vi "Initialize Root.vi"(6 "RootQueueName":string, 8 "error in (no error)":errorcluster caption="错误输入（无错误）", 9 "CurrentVi*":refnum<vi>, 10 "RootPanel*":refnum<vi>, 11 "PanelRootNode 输入":refnum<class "PanelRootNode.lvclass"> caption="DNL_LabVIEW Object in") -> (0 "error out":errorcluster caption="错误输出", 2 "SelfNode*":refnum<data-value>)   [LabVIEW 2013, in "PanelRootNode.lvclass"]
uses:
  PanelRootNode.lvclass
  PanelRootNode.lvclass/PanelRootNode.ctl
  PanelDataNode/PanelDataNode.lvclass/PanelDataNode.ctl
  PanelDataNode/PanelDataNode.lvclass
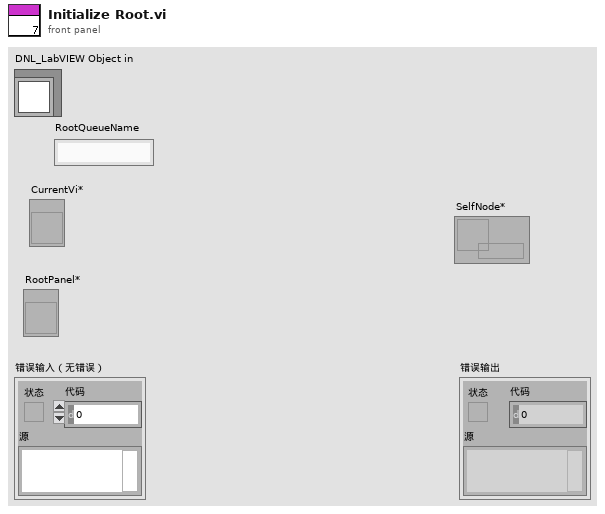
[diagram p1: front panel]
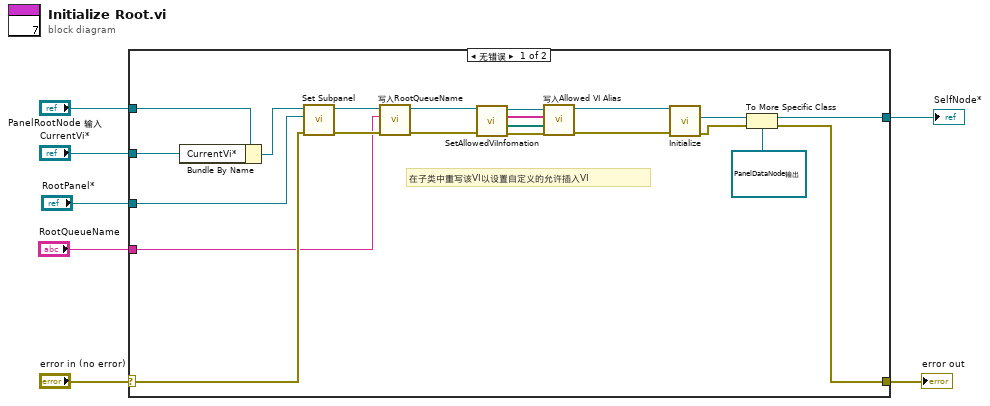
[diagram p0: block diagram]
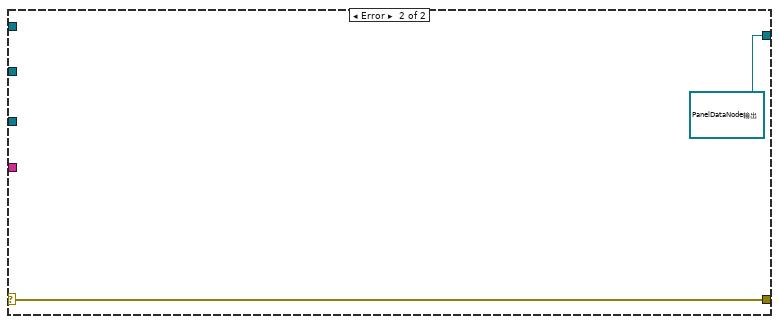
[diagram p2: hidden frame]
diagram:
  n1 = case shown="无错误" "error in (no error)" {
    selector: "error in (no error)" -> [w18 w30]
    tunnel: [w19 w30] -> w6
    tunnel: "PanelRootNode 输入" -> [w25 _]
    tunnel: "RootPanel*" -> [w28 _]
    tunnel: [w16 refnum<data-value> refnum ("data value reference")] -> w3
    tunnel: "CurrentVi*" -> [w21 _]
    tunnel: "RootQueueName" -> [w17 _]
    frame No Error {
      # "在子类中重写该VI以设置自定义的允许插入VI"
      n2 = Bundle By Name(cluster=w25, "CurrentVi*"=w21) -> (w24:refnum<class "PanelRootNode.lvclass">)
      n3 = call "Set Subpanel.vi"("error in (no error)"=w18, "Subpanel*"=w28, "PanelDataNode输入"=w24) -> ("error out"=w23:errorcluster, "PanelDataNode输出"=w22:refnum<class "PanelRootNode.lvclass">)  [unwired: 7 in]
      n4 = call "写入RootQueueName.vi"("error in (no error)"=w23, "RootQueueName"=w17, "PanelDataNode输入"=w22) -> ("error out"=w14:errorcluster, "PanelDataNode输出"=w15:refnum<class "PanelRootNode.lvclass">)  [unwired: 7 in]
      n5 = call-dynamic "SetAllowedViInfomation.vi"("error in (no error)"=w14, "PanelRootNode 输入"=w15) -> ("error out"=w10:errorcluster, "ViPath"=w11:path[], "ViAlias"=w12:string[], "PanelRootNode 输出"=w13:refnum<class "PanelRootNode.lvclass">)  [unwired: 6 in]
      n6 = call "写入Allowed VI Alias.vi"("error in (no error)"=w10, "Allowed VI Path"=w11, "Allowed VI Alias"=w12, "PanelDataNode输入"=w13) -> ("error out"=w8:errorcluster, "PanelDataNode输出"=w9:refnum<class "PanelRootNode.lvclass">)  [unwired: 6 in]
      n7 = call-dynamic "Initialize.vi"("error in"=w8, "PanelRootNode in"=w9) -> ("error out"=w20:errorcluster, "SelfNode*"=w27:refnum<data-value>)  [unwired: 7 in]
      n8 = To More Specific Class(target class=refnum<data-value> refnum ("数据值引用"), reference=w27, error in=w20) -> (specific class reference=w16:refnum<data-value>, error out=w19:errorcluster)
    }
    frame Error {
    }
  }
  "error out" <- w6
  "SelfNode*" <- w3
